vi "choose bandpass filter.vi"(3 "color table":i32[](array[numeric]), 4 "Cal image data":dbl[][](array[numeric]), 5 "Power spectrum":dbl[](array[numeric]), 6 "?":string) -> (0 "forget radius":i32=10, 1 "High bandpass":i32, 2 "Low bandpass":i32)   [LabVIEW 2014]
uses:
  <vilib>/Analysis/2dsp.llb/Real FFT.vi
  <vilib>/Analysis/2dsp.llb/Inverse Complex FFT.vi
  <vilib>/picture/picture.llb/Draw 8-Bit Pixmap.vi
  <vilib>/Analysis/NI_AALPro.lvlib
panel:
  out "input forget":i32
  out "phi vs z":dbl[](graph)
  out "delta phi vs z":dbl[](graph)
  out "?":string
  out "Cal image with chosen filter":picture
  out "Cal image":picture
  out "stop 2":bool
  in  "Click here when done":bool
  out "Averaged Power Spectrum":dbl[](graph)
  # "Drag cursors to bracket the bandpass region for Hilbert filtering"
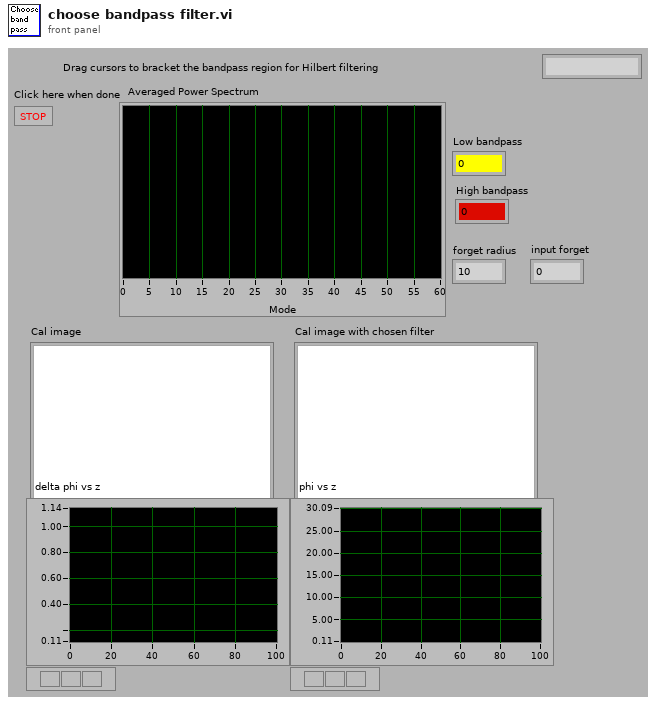
[diagram p1: front panel]
types:
  T1 = cluster{"[0]":i32, "[1]":i32, "[2]":i32, "[3]":i32}
  T2 = typedef "LVMouseTypeDef.ctl" = cluster{"Mouse Position":cluster{"X":i32, "Y":i32}, "Mouse Modifiers":cluster{"Button Down":bool, "Shift Mod":bool, "Menu Mod":bool, "Option Mod":bool}}
  T3 = typedef "LVCursorListTypeDef.ctl" = cluster{"Name":string, "Color":u32, "Style":u8, "Point Style":u8, "Name Visible":bool, "Allow Drag":bool, "Cursor Mode":u32, "Plot":i32, "Index":i32, "Position":cluster{"X":dbl, "Y":dbl}, "X Scale":u32, "Y Scale":u32, "Watch Plots":i32[], "Watch All Plots":bool, "Plot Area":i32, "Label Offset":cluster{"X":dbl, "Y":dbl}}[]
  T4 = cluster{"Name":string, "Color":u32, "Style":u8, "Point Style":u8, "Name Visible":bool, "Allow Drag":bool, "Cursor Mode":u32, "Plot":i32, "Index":i32, "Position":cluster{"X":dbl, "Y":dbl}, "X Scale":u32, "Y Scale":u32, "Watch Plots":i32[], "Watch All Plots":bool, "Plot Area":i32, "Label Offset":cluster{"X":dbl, "Y":dbl}}
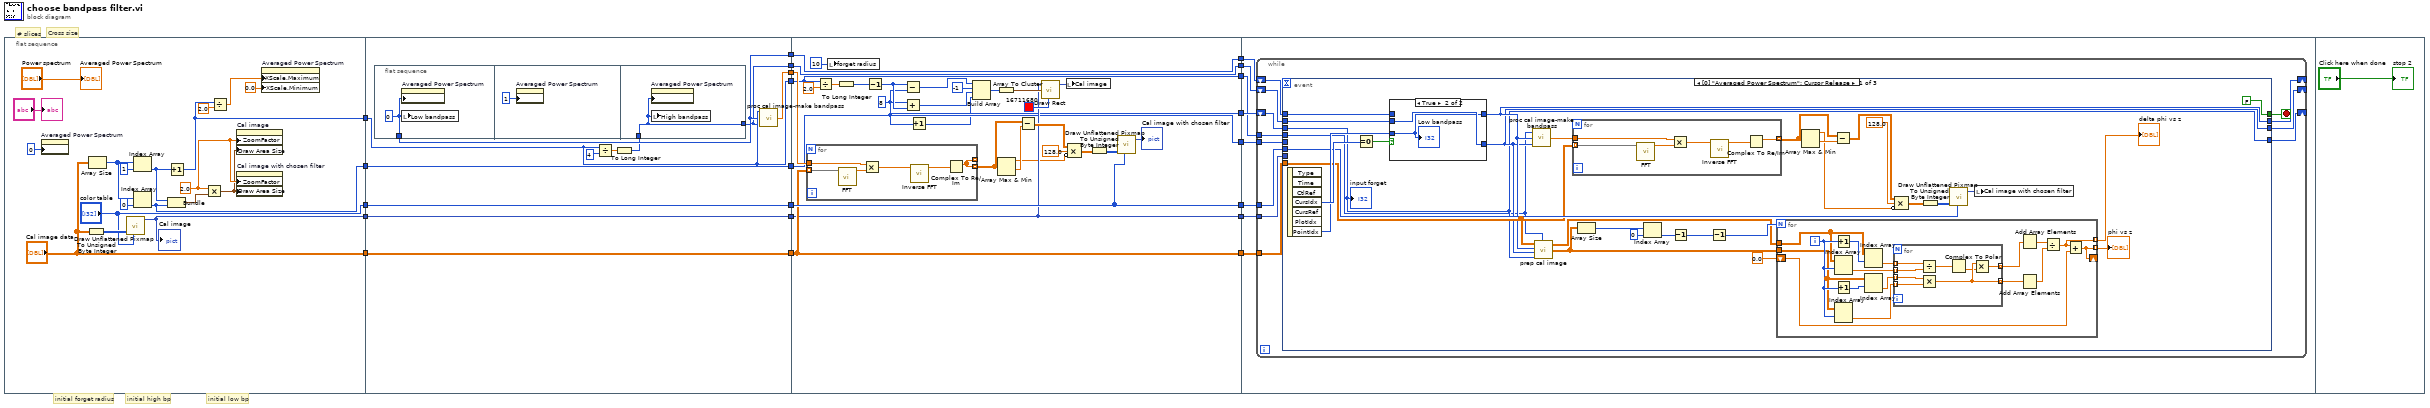
[diagram p0: block diagram]
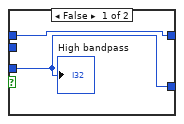
[diagram p2: hidden frame]
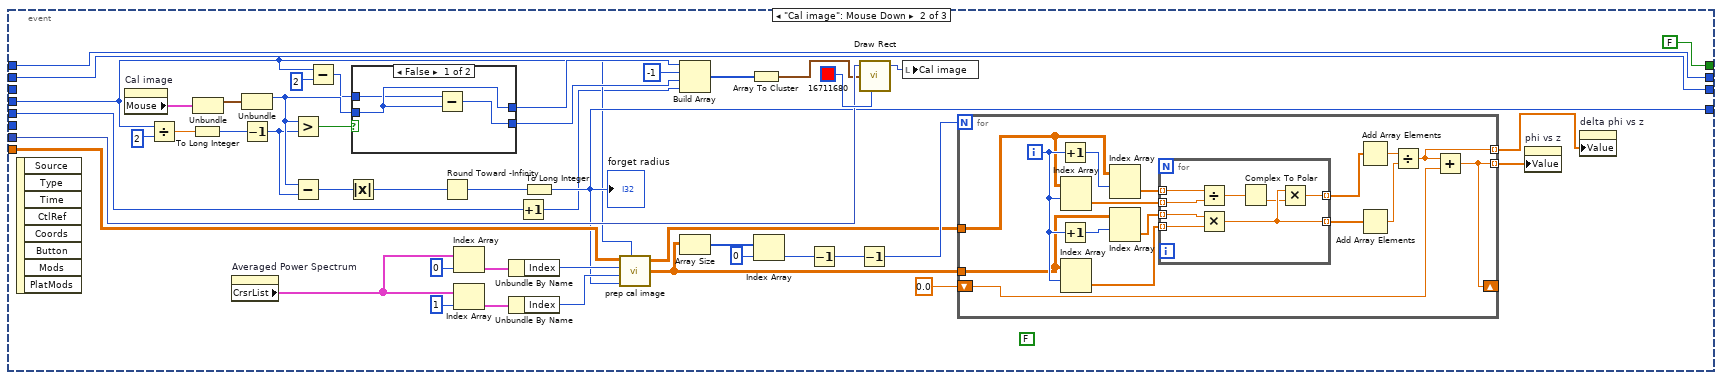
[diagram p3: hidden frame]
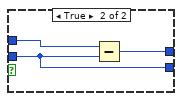
[diagram p4: hidden frame]
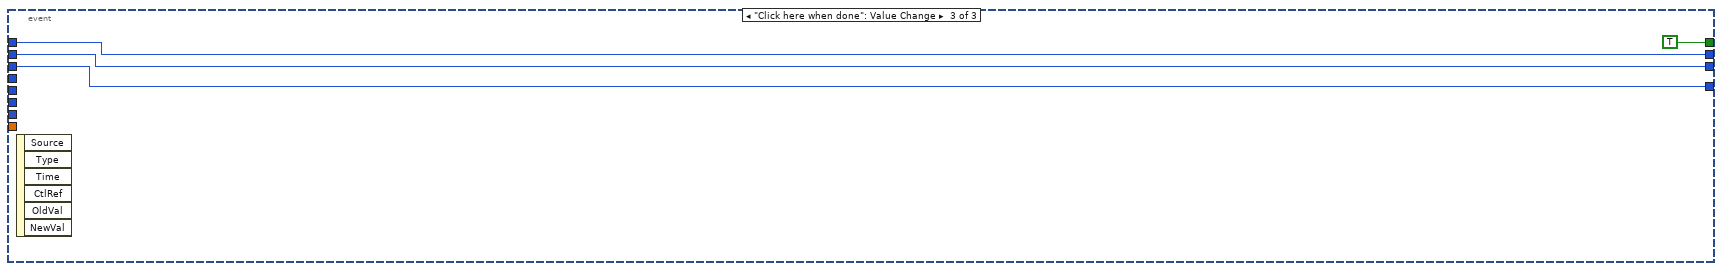
[diagram p5: hidden frame]
diagram:
  # "# slices"
  # "initial forget radius"
  # "initial high bp"
  # "initial low bp"
  # "Cross size"
  n1 = flat-sequence {
    tunnel: ["Cal image data"] -> w21
    tunnel: ["color table"] -> w20
    tunnel: [w37] -> w19
    tunnel: [w30] -> w18
    tunnel: [w22] -> w17
    tunnel: w21 -> [w44]
    tunnel: [w44] -> w16
    tunnel: w20 -> [w43]
    tunnel: [w43] -> w15
    tunnel: w19 -> [w42]
    tunnel: [w42] -> w14
    tunnel: w18 -> [w49]
    tunnel: [w49] -> w13
    tunnel: [w45] -> w12
    tunnel: [w48] -> w11
    tunnel: [w47] -> w10
    tunnel: w17 -> [w41]
    tunnel: [w41] -> w9
    tunnel: w16 -> [w72]
    tunnel: [w72] -> w8
    tunnel: w15 -> [w83]
    tunnel: [w83] -> w7
    tunnel: w14 -> [w71]
    tunnel: [w71] -> w6
    tunnel: w13 -> [w63]
    tunnel: [w63] -> w5
    tunnel: w12 -> [w67]
    tunnel: w11 -> [w58]
    tunnel: [w58] -> w4
    tunnel: w10 -> [w57]
    tunnel: [w57] -> w3
    tunnel: [w61] -> w2
    tunnel: w9 -> [w60]
    tunnel: [w60] -> w1
    tunnel: w8 -> [w97]
    tunnel: w7 -> [w98]
    tunnel: w6 -> [w96]
    tunnel: w5 -> [w92]
    tunnel: w4 -> [w95]
    tunnel: w3 -> [w94]
    tunnel: w2 -> [w93]
    tunnel: w1 -> [w91]
    frame #0 {
      w25 = sgl 2.0 ("Zoom Factor")
      n2 = property on="Averaged Power Spectrum" class="WFGraph (strict)"("Active Cursor"=u32 0) -> ()  [unwired: 2 in, 2 out]
      n3 = To Unsigned Byte Integer(number="Cal image data") -> (unsigned 8bit integer=w39:u8[][])
      n4 = Array Size(array="Cal image data") -> (size(s)=w28:i32[])
      n5 = call-poly <vilib>:"Draw Unflattened Pixmap.vi"("data"=w39, "color table"="color table") -> ("new picture"=w37:picture)  [unwired: 7 in]
      "Cal image" <- w37
      n6 = Index Array(array=w28, index=1) -> (element=w26:i32)
      n7 = Index Array(array=w28, index=0) -> (element=w22:i32)
      n8 = Bundle(w26, w22) -> (w24:cluster{i32, i32})  [unwired: 1 in]
      n9 = Increment(x=w26) -> (x+1=w30:i32)
      n10 = Multiply(x=w25, y=w24) -> (x*y=w23:cluster{sgl, sgl})
      n11 = Divide(x=w30, y=2.0) -> (x/y=w29:dbl)
      n12 = property on="Cal image" class="Pict"("ZoomFactor"=w25, "Draw Area Size"=w23) -> ()  [unwired: 2 in, 2 out]
      n13 = property on="Cal image with chosen filter" class="Pict"("ZoomFactor"=w25, "Draw Area Size"=w23) -> ()  [unwired: 2 in, 2 out]
      n14 = property on="Averaged Power Spectrum" class="WFGraph (strict)"("XScale.Maximum"=w29, "XScale.Minimum"=0.0 ("X Scale.Range:Minimum")) -> ()  [unwired: 2 in, 2 out]
      "Averaged Power Spectrum" <- "Power spectrum"
      "?" <- "?"
    }
    frame #1 {
      n15 = flat-sequence {
        tunnel: [w52] -> w48
        tunnel: w46 -> [w54]
        tunnel: [w54] -> w47
        frame #0 {
          w52 = 0 ("Cursor.Cursor Index")
          n16 = property on="Averaged Power Spectrum" class="WFGraph (strict)"("Cursor.Cursor Index"=w52) -> ()  [unwired: 2 in, 2 out]
          n17 = local write "Low bandpass"(w52) -> ()
        }
        frame #1 {
          n18 = property on="Averaged Power Spectrum" class="WFGraph (strict)"("Active Cursor"=u32 1) -> ()  [unwired: 2 in, 2 out]
        }
        frame #2 {
          n19 = property on="Averaged Power Spectrum" class="WFGraph (strict)"("Cursor.Cursor Index"=w54) -> ()  [unwired: 2 in, 2 out]
          n20 = local write "High bandpass"(w54) -> ()
        }
      }
      n21 = Divide(x=w49, y=4) -> (x/y=w50:dbl)
      n22 = To Long Integer(number=w50) -> (32bit integer=w46:i32)
      n23 = call "proc cal image-make bandpass.vi"("HIGH bandpass\n(mode)"=w47, "LOW bandpass\n(mode)"=w48, "# of points (cross size)"=w49) -> ("Cosine bandpass"=w45:sgl[])
    }
    frame #2 {
      w61 = 8 ("x")
      n24 = for {
        tunnel: w67 -> [w89]
        tunnel: [w85] -> _ mode=indexing
        tunnel: w72 -> [w86] mode=indexing
        tunnel: [w85] -> w80 mode=indexing
        n25 = call-poly <vilib>:"FFT.vi"("X"=w86) -> ("FFT {X}"=w90:cdb[])  [unwired: 9 in, 1 out]
        n26 = Multiply(x=w89, y=w90) -> (x*y=w88:cdb[])
        n27 = call-poly <vilib>:"Inverse FFT.vi"("FFT {X}"=w88) -> ("X"=w87:cdb[])  [unwired: 9 in, 1 out]
        n28 = Complex To Re/Im(x + iy=w87) -> (x=w85:dbl[])  [unwired: 1 out]
      }
      n29 = Divide(x=w63, y=2.0) -> (x/y=w65:dbl)
      n30 = local write "forget radius"(10 ("x")) -> ()
      n31 = To Long Integer(number=w65) -> (32bit integer=w64:i32)
      n32 = Decrement(x=w64) -> (x-1=w62:i32)
      n33 = Subtract(x=w62, y=w61) -> (x-y=w70:i32)
      n34 = Add(x=w61, y=w62) -> (x+y=w69:i32)
      n35 = Increment(x=w60) -> (x+1=w59:i32)
      n36 = Build Array(w70, -1 ("# of points (cross size)"), w69, w59) -> (w74:i32[])
      n37 = Array To Cluster(array=w74) -> (cluster=w75:T1)
      n38 = Array Max & Min(array=w80) -> (max value=w55:dbl, min value=w56:dbl)  [unwired: 2 out]
      n39 = Subtract(x=w80, y=w56) -> (x-y=w81:dbl[][])
      n40 = call <vilib>:"Draw Rect.vi"("picture"=w71, "rect"=w75, "color(black)"=u32 16711680) -> ("new picture"=w73:picture)  [unwired: 6 in]
      n41 = local write "Cal image"(w73) -> ()
      n42 = Compound Arithmetic op=MULTIPLY(w81, 128.0 ("value"), invert w55) -> (w79:dbl[][])
      n43 = To Unsigned Byte Integer(number=w79) -> (unsigned 8bit integer=w78:u8[][])
      n44 = call-poly <vilib>:"Draw Unflattened Pixmap.vi"("data"=w78, "color table"=w83) -> ("new picture"=→"Cal image with chosen filter":picture)  [unwired: 7 in]
    }
    frame #3 {
      n45 = while {
        shift-right: [w106] -> _
        shift-left: w95 -> [w109]
        shift-right: [w105] -> _
        shift-left: w94 -> [w108]
        tunnel: w97 -> [w107]
        tunnel: w98 -> [w104]
        tunnel: w96 -> [w103]
        shift-right: [w102] -> _
        shift-left: w93 -> [w101]
        tunnel: w92 -> [w100]
        tunnel: w91 -> [w99]
        stop <- w110 stop-if-true
        n46 = event shown="[0] \"Averaged Power Spectrum\": Cursor Release" {
          selector: _ -> [_ _ _]
          dyn-events: _ -> [_ _ _]
          timeout: _ -> [_ _ _]
          tunnel: [FALSE FALSE TRUE] -> w110
          tunnel: w109 -> [w137 w205 w254]
          tunnel: w108 -> [w136 w204 w253]
          tunnel: w107 -> [w122 w192 _]
          tunnel: [w121 w205 w254] -> w106
          tunnel: [w120 w204 w253] -> w105
          tunnel: w104 -> [w132 _ _]
          tunnel: w99 -> [_ w212 _]
          tunnel: w103 -> [_ w210 _]
          tunnel: [w112 w184 w252] -> w102
          tunnel: w101 -> [w112 _ w252]
          tunnel: w100 -> [w111 w179 _]
          event "Averaged Power Spectrum": Cursor Release {
            n47 = event-data() -> ("CursIdx"=w141:i32, "PointIdx"=w139:i32)  [unwired: 1 in, 5 out]
            n48 = Equal To 0?(x=w141) -> (x = 0?=w140:bool)
            n49 = case shown="True" w140 {
              tunnel: w139 -> [w172 w174]
              tunnel: w137 -> [w173 _]
              tunnel: w136 -> [_ w175]
              tunnel: [w172 w175] -> w120
              tunnel: [w173 w174] -> w121
              frame False {
                "High bandpass" <- w172
              }
              frame True {
                "Low bandpass" <- w174
              }
            }
            n50 = call "proc cal image-make bandpass.vi"("HIGH bandpass\n(mode)"=w120, "LOW bandpass\n(mode)"=w121, "# of points (cross size)"=w111) -> ("Cosine bandpass"=w133:sgl[])
            n51 = call "prep cal image.vi"("Raw cal image"=w122, "LOW bandpass\n(mode)"=w121, "HIGH bandpass\n(mode)"=w120, "forget radius"=w112, "# of points (cross size)"=w111) -> ("r-shifted corkscrew cal"=w119:cdb[][], "r shifted cal ampl"=w118:dbl[][])  [unwired: 1 out]
            n52 = for {
              tunnel: [w167] -> w126 mode=indexing
              tunnel: w122 -> [w169] mode=indexing
              tunnel: w133 -> [w168]
              n53 = call-poly <vilib>:"FFT.vi"("X"=w169) -> ("FFT {X}"=w171:cdb[])  [unwired: 9 in, 1 out]
              n54 = Multiply(x=w168, y=w171) -> (x*y=w170:cdb[])
              n55 = call-poly <vilib>:"Inverse FFT.vi"("FFT {X}"=w170) -> ("X"=w166:cdb[])  [unwired: 9 in, 1 out]
              n56 = Complex To Re/Im(x + iy=w166) -> (x=w167:dbl[])  [unwired: 1 out]
            }
            n57 = Array Size(array=w118) -> (size(s)=w117:i32[])
            n58 = Index Array(array=w117, index=0) -> (element=w116:i32)
            n59 = Decrement(x=w116) -> (x-1=w114:i32)
            n60 = Decrement(x=w114) -> (x-1=w125:i32)
            n61 = for {
              N: w125 -> [_]
              tunnel: [w144] -> w124 mode=indexing
              tunnel: w118 -> [w150]
              tunnel: w119 -> [w149]
              shift-right: [w142] -> _
              shift-left: 0.0 -> [w143]
              tunnel: [w142] -> w113 mode=indexing
              i -> [w153]
              n62 = Increment(x=w153) -> (x+1=w152:i32)
              n63 = Index Array(array=w149, index (row)=w153) -> (element=w145:cdb[])  [unwired: 1 in]
              n64 = Increment(x=w153) -> (x+1=w151:i32)
              n65 = Index Array(array=w150, index (row)=w153) -> (element=w147:dbl[])  [unwired: 1 in]
              n66 = Index Array(array=w149, index (row)=w152) -> (element=w146:cdb[])  [unwired: 1 in]
              n67 = Index Array(array=w150, index (row)=w151) -> (element=w148:dbl[])  [unwired: 1 in]
              n68 = for {
                tunnel: w146 -> [w160] mode=indexing
                tunnel: w148 -> [w165] mode=indexing
                tunnel: w147 -> [w164] mode=indexing
                tunnel: w145 -> [w161] mode=indexing
                tunnel: [w163] -> w156 mode=indexing
                tunnel: [w162] -> w157 mode=indexing
                n69 = Divide(x=w160, y=w161) -> (x/y=w159:cdb)
                n70 = Multiply(x=w165, y=w164) -> (x*y=w162:dbl)
                n71 = Complex To Polar(r * e^(i*theta)=w159) -> (theta=w158:dbl)  [unwired: 1 out]
                n72 = Multiply(x=w162, y=w158) -> (x*y=w163:dbl)
              }
              n73 = Add Array Elements(numeric array=w156) -> (sum=w155:dbl)
              n74 = Add Array Elements(numeric array=w157) -> (sum=w154:dbl)
              n75 = Divide(x=w155, y=w154) -> (x/y=w144:dbl)
              n76 = Add(x=w144, y=w143) -> (x+y=w142:dbl)
            }
            "delta phi vs z" <- w124
            "phi vs z" <- w113
            n77 = Array Max & Min(array=w126) -> (max value=w130:dbl, min value=w131:dbl)  [unwired: 2 out]
            n78 = Subtract(x=w126, y=w131) -> (x-y=w128:dbl[][])
            n79 = Compound Arithmetic op=MULTIPLY(w128, 128.0 ("value"), invert w130) -> (w127:dbl[][])
            n80 = To Unsigned Byte Integer(number=w127) -> (unsigned 8bit integer=w135:u8[][])
            n81 = call-poly <vilib>:"Draw Unflattened Pixmap.vi"("data"=w135, "color table"=w132) -> ("new picture"=w134:picture)  [unwired: 7 in]
            n82 = local write "Cal image with chosen filter"(w134) -> ()
            "input forget" <- w112
          }
          event "Cal image": Mouse Down {
            (unwired) FALSE
            n83 = event-data() -> ()  [unwired: 1 in, 8 out]
            n84 = property on="Cal image" class="Pict"() -> ("Mouse"=w218:T2)  [unwired: 2 in, 2 out]
            n85 = Divide(x=w179, y=2) -> (x/y=w182:dbl)
            n86 = To Long Integer(number=w182) -> (32bit integer=w181:i32)
            n87 = Unbundle(w218) -> ("Mouse Position"=w217:cluster{"X":i32, "Y":i32})  [unwired: 1 out]
            n88 = property on="Averaged Power Spectrum" class="WFGraph (strict)"() -> ("CrsrList"=w191:T3)  [unwired: 2 in, 2 out]
            n89 = Unbundle(w217) -> ("X"=w203:i32)  [unwired: 1 out]
            n90 = Decrement(x=w181) -> (x-1=w180:i32)
            n91 = Greater?(x=w203, y=w180) -> (0:w216:bool)
            n92 = Subtract(x=w203, y=w180) -> (x-y=w221:i32)
            n93 = Subtract(x=w179, y=2) -> (x-y=w177:i32)
            n94 = Absolute Value(x=w221) -> (abs(x)=w220:i32)
            n95 = case shown="False" w216 {
              tunnel: w203 -> [w248 w250]
              tunnel: [w248 w251] -> w215
              tunnel: [w247 w250] -> w213
              tunnel: w177 -> [w246 w249]
              frame False {
                n96 = Subtract(x=w246, y=w248) -> (x-y=w247:i32)
              }
              frame True {
                n97 = Subtract(x=w249, y=w250) -> (x-y=w251:i32)
              }
            }
            n98 = Round Toward -Infinity(1:w220) -> (0:w219:i32)
            n99 = Index Array(array=w191, index=0) -> (element=w188:T4)
            n100 = Index Array(array=w191, index=1) -> (element=w187:T4)
            n101 = Unbundle By Name(w188) -> ("Index"=w186:i32)
            n102 = Unbundle By Name(w187) -> ("Index"=w185:i32)
            n103 = Increment(x=w212) -> (x+1=w176:i32)
            n104 = To Long Integer(number=w219) -> (32bit integer=w184:i32)
            "forget radius" <- w184
            n105 = call "prep cal image.vi"("Raw cal image"=w192, "LOW bandpass\n(mode)"=w186, "HIGH bandpass\n(mode)"=w185, "forget radius"=w184, "# of points (cross size)"=w179) -> ("r-shifted corkscrew cal"=w200:cdb[][], "r shifted cal ampl"=w199:dbl[][])  [unwired: 1 out]
            n106 = Build Array(w215, -1 ("# of points (cross size)"), w213, w176) -> (w206:i32[])
            n107 = Array Size(array=w199) -> (size(s)=w198:i32[])
            n108 = Array To Cluster(array=w206) -> (cluster=w208:T1)
            n109 = Index Array(array=w198, index=0) -> (element=w197:i32)
            n110 = Decrement(x=w197) -> (x-1=w195:i32)
            n111 = Decrement(x=w195) -> (x-1=w202:i32)
            n112 = call <vilib>:"Draw Rect.vi"("picture"=w210, "rect"=w208, "color(black)"=u32 16711680) -> ("new picture"=w209:picture)  [unwired: 6 in]
            n113 = local write "Cal image"(w209) -> ()
            n114 = for {
              N: w202 -> [_]
              tunnel: [w224] -> w194 mode=indexing
              tunnel: w199 -> [w230]
              tunnel: w200 -> [w229]
              shift-right: [w222] -> _
              shift-left: 0.0 -> [w223]
              tunnel: [w222] -> w193 mode=indexing
              i -> [w233]
              n115 = Increment(x=w233) -> (x+1=w232:i32)
              n116 = Increment(x=w233) -> (x+1=w231:i32)
              n117 = Index Array(array=w229, index (row)=w233) -> (element=w225:cdb[])  [unwired: 1 in]
              n118 = Index Array(array=w230, index (row)=w233) -> (element=w227:dbl[])  [unwired: 1 in]
              n119 = Index Array(array=w229, index (row)=w232) -> (element=w226:cdb[])  [unwired: 1 in]
              n120 = Index Array(array=w230, index (row)=w231) -> (element=w228:dbl[])  [unwired: 1 in]
              n121 = for {
                tunnel: w226 -> [w240] mode=indexing
                tunnel: w228 -> [w245] mode=indexing
                tunnel: w227 -> [w244] mode=indexing
                tunnel: w225 -> [w241] mode=indexing
                tunnel: [w243] -> w236 mode=indexing
                tunnel: [w242] -> w237 mode=indexing
                n122 = Divide(x=w240, y=w241) -> (x/y=w239:cdb)
                n123 = Multiply(x=w245, y=w244) -> (x*y=w242:dbl)
                n124 = Complex To Polar(r * e^(i*theta)=w239) -> (theta=w238:dbl)  [unwired: 1 out]
                n125 = Multiply(x=w242, y=w238) -> (x*y=w243:dbl)
              }
              n126 = Add Array Elements(numeric array=w236) -> (sum=w235:dbl)
              n127 = Add Array Elements(numeric array=w237) -> (sum=w234:dbl)
              n128 = Divide(x=w235, y=w234) -> (x/y=w224:dbl)
              n129 = Add(x=w224, y=w223) -> (x+y=w222:dbl)
            }
            n130 = property on="phi vs z" class="WFGraph (strict)"("Value"=w193) -> ()  [unwired: 2 in, 2 out]
            n131 = property on="delta phi vs z" class="WFGraph (strict)"("Value"=w194) -> ()  [unwired: 2 in, 2 out]
          }
          event "Click here when done": Value Change {
            n132 = event-data() -> ()  [unwired: 1 in, 6 out]
          }
        }
      }
    }
    frame #4 {
      "stop 2" <- "Click here when done"
    }
  }
